vi "Credentials Grant.vi"(4 "client secret":string, 6 "client id":string, 7 "token request uri":string, 8 "error in (no error)":errorcluster, 9 "password":string, 10 "username":string, 11 "grant_type":string) -> (0 "error out":errorcluster, 3 "token response (JSON)":string)   [LabVIEW 2020, in "Netatmo-WeatherStation.lvlib"]
uses:
  Netatmo-WeatherStation.lvlib
  <vilib>/httpClient/POSTBuffer.vi
  <vilib>/httpClient/LabVIEWHTTPClient.lvlib
panel:
  in  "scope":string="read_station"
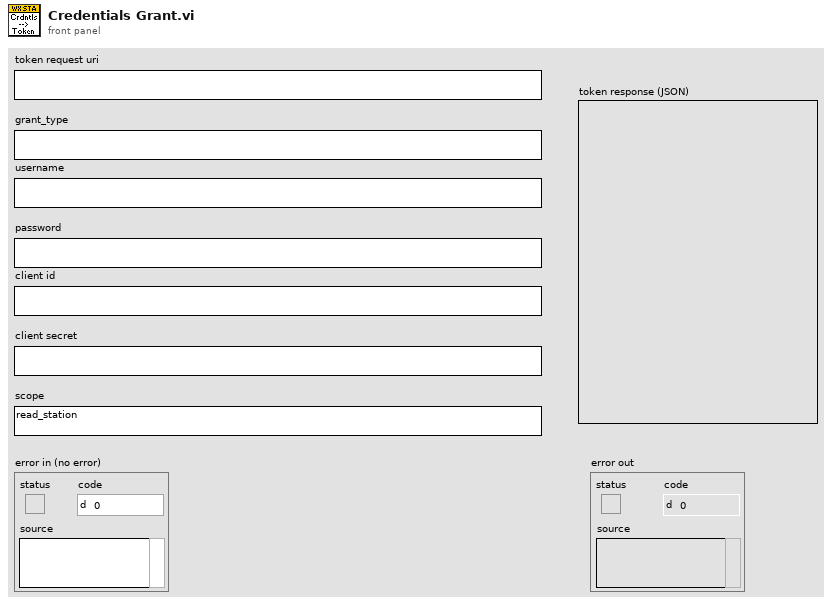
[diagram p1: front panel]
types:
  T1 = typedef "LabVIEWHTTPClient.lvlib/ClientHandle.ctl" = refnum<k1>
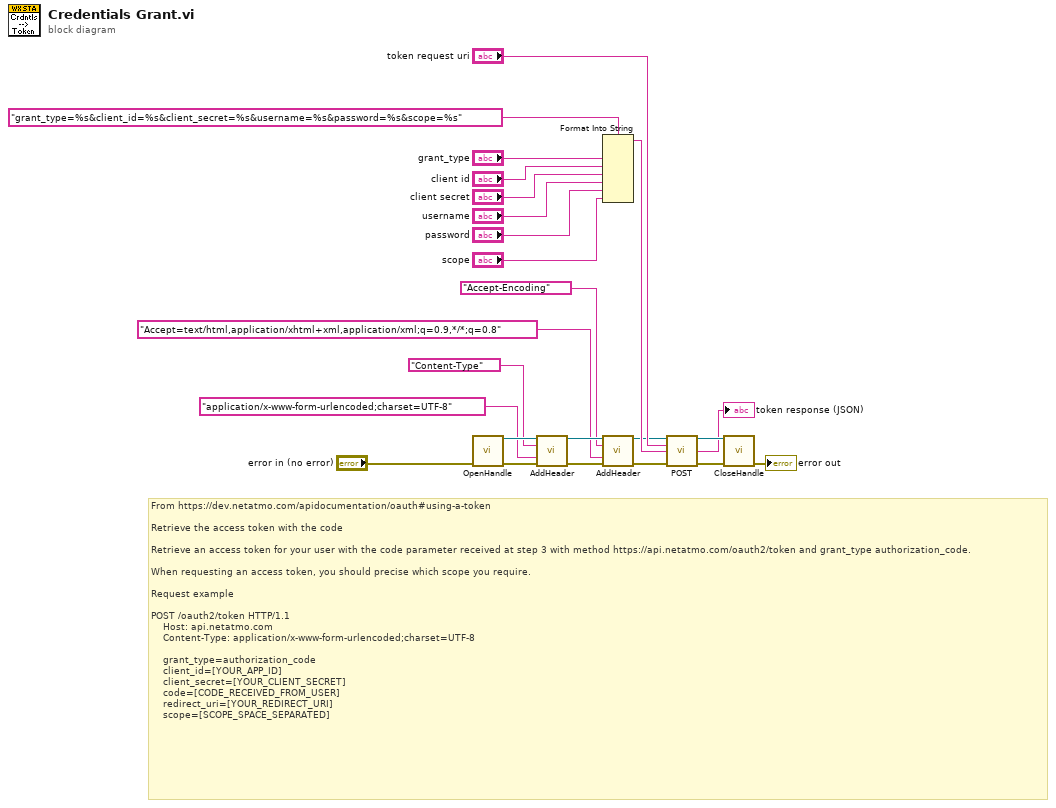
[diagram p0: block diagram]
diagram:
  # "From https://dev.netatmo.com/apidocumentation/oauth#using-a-token\n\nRetrieve the access token with the code\n\nRetrieve an access token for your user with the code parameter received at step 3 with method https://api.netatmo.com/oauth2/token and grant_type authorization_code.\n\nWhen requesting an access token, you should precise which scope you require.\n\nRequest example\n\nPOST /oauth2/token HTTP/1.1\n    Host: api.netatmo.com\n    Content-Type: application/x-www-form-urlencoded;charset=UTF-8\n\n    grant_type=authorization_code\n    client_id=[YOUR_APP_ID]\n    client_secret=[YOUR_CLIENT_SECRET]\n    code=[CODE_RECEIVED_FROM_USER]\n    redirect_uri=[YOUR_REDIRECT_URI]\n    scope=[SCOPE_SPACE_SEPARATED]"
  n1 = call <vilib>:"OpenHandle.vi"("error in (no error)"="error in (no error)") -> ("client handle out"=w23:T1, "error out"=w17:errorcluster)  [unwired: 13 in]
  n2 = call <vilib>:"AddHeader.vi"("client handle"=w23, "header"="Content-Type", "value"="application/x-www-form-urlencoded;charset=UTF-8", "error in (no error)"=w17) -> ("client handle out"=w20:T1, "error out"=w16:errorcluster)  [unwired: 10 in]
  n3 = Format Into String(format string="grant_type=%s&client_id=%s&client_secret=%s&username=%s&password=%s&scope=%s", "grant_type", "client id", "client secret", "username", "password", "scope") -> (resulting string=w14:string)  [unwired: 2 in, 1 out]
  n4 = call <vilib>:"AddHeader.vi"("client handle"=w20, "header"="Accept-Encoding", "value"="Accept=text/html,application/xhtml+xml,application/xml;q=0.9,*/*;q=0.8", "error in (no error)"=w16) -> ("client handle out"=w13:T1, "error out"=w12:errorcluster)  [unwired: 10 in]
  n5 = call-poly <vilib>:"POST.vi"("client handle"=w13, "url"="token request uri", "buffer"=w14, "error in (no error)"=w12) -> ("client handle out"=w11:T1, "body"=→"token response (JSON)":string, "error out"=w10:errorcluster)  [unwired: 8 in, 1 out]
  n6 = call <vilib>:"CloseHandle.vi"("client handle"=w11, "error in (no error)"=w10) -> ("error out"=→"error out":errorcluster)  [unwired: 13 in]
